vi "Instruction Set Test.vi"(11 "CPUFail":bool) -> (0 "error out":errorcluster, 3 "Result":bool)   [LabVIEW 2025]
doc: "Verifies that sample instruction sets are correctly executed by the CPU."
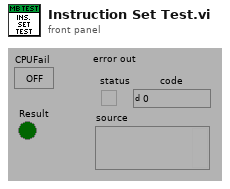
[diagram p1: front panel]
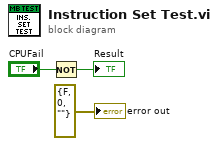
[diagram p0: block diagram]
diagram:
  n1 = Not(x="CPUFail") -> (.not. x?=→"Result":bool)
  "error out" <- errorcluster {"status"=FALSE, "code"=0, "source"=""} ("error out")
